vi "Get Display Text.vi"(8 "error in (no error)":errorcluster, 11 "Element Array in":refnum<class "Element Array.lvclass">) -> (0 "error out":errorcluster, 1 "Detail Text":string, 2 "Display Name":string, 3 "Element Array out":refnum<class "Element Array.lvclass">)   [LabVIEW 2023, in "VILab.lvlib" / "Element Array.lvclass"]
uses:
  Element Array.lvclass
  Element Array.lvclass/Element Array.ctl
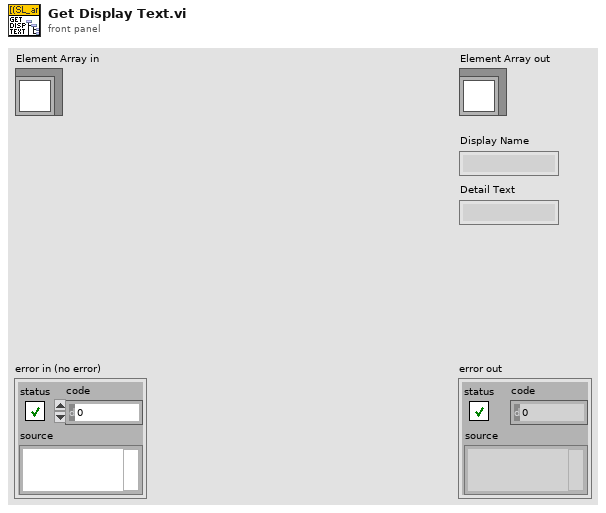
[diagram p1: front panel]
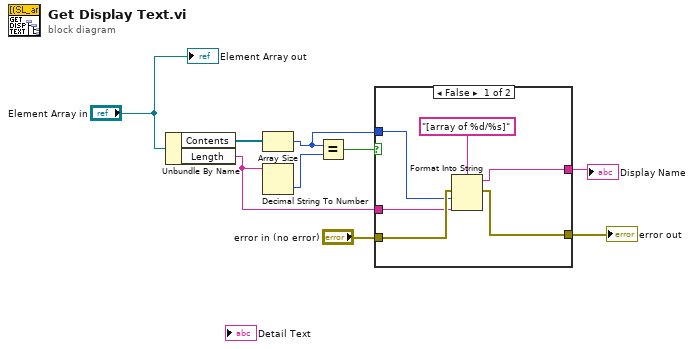
[diagram p0: block diagram]
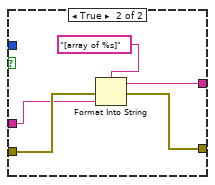
[diagram p2: hidden frame]
diagram:
  n1 = Unbundle By Name("Element Array in") -> ("Contents"=w8:refnum<class "Attribute.lvclass">[], "Length"=w3:string)
  n2 = Array Size(array=w8) -> (size(s)=w1:i32)
  n3 = Decimal String To Number(string=w3) -> (number=w7:i32)  [unwired: 2 in, 1 out]
  n4 = Equal?(x=w1, y=w7) -> (x = y?=w6:bool)
  n5 = case shown="False" w6 {
    tunnel: "error in (no error)" -> [w13 w20]
    tunnel: [w12 w19] -> w4
    tunnel: w3 -> [w11 w18]
    tunnel: [w14 w16] -> w2
    tunnel: w1 -> [w10 _]
    frame False {
      n6 = Format Into String(format string="[array of %d/%s]", error in=w13, w10, w11) -> (resulting string=w14:string, error out=w12:errorcluster)  [unwired: 1 in]
    }
    frame True {
      n7 = Format Into String(format string="[array of %s]", error in=w20, w18) -> (resulting string=w16:string, error out=w19:errorcluster)  [unwired: 1 in]
    }
  }
  "error out" <- w4
  "Display Name" <- w2
  "Element Array out" <- "Element Array in"
